vi "_Read.vi"(8 "error in (no error)":errorcluster, 11 "Synapse CCD in":refnum<class "Synapse CCD.lvclass">) -> (0 "error out":errorcluster, 2 "X array":T1, 3 "Synapse CCD out":refnum<class "Synapse CCD.lvclass">)   [LabVIEW 2012, in "Synapse CCD.lvclass"]
doc: "(Protected, Dynamic, Pure Virtual/Abstract) Perform a measurement and return one or more channels of data. Outsiders should not call this method, but instead the public \"Read Data.vi\"."
uses:
  Synapse CCD.lvclass
  Utility Classes/Readable/X array.ctl
  Utility Classes/Readable/X.ctl
  Utility Classes/Readable/Readable.lvclass
  Synapse CCD.lvclass/Synapse CCD.ctl
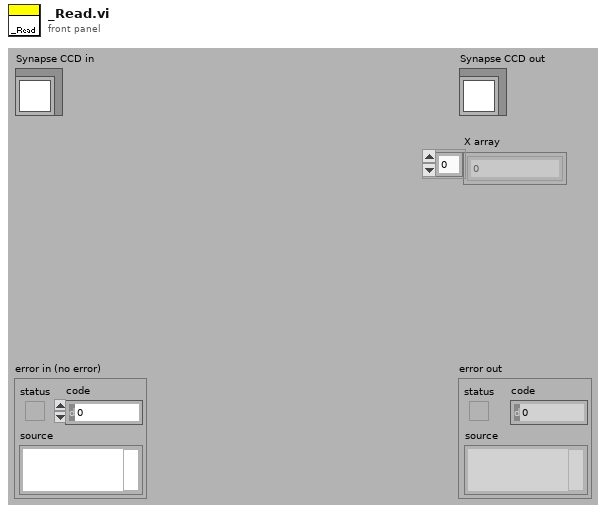
[diagram p1: front panel]
types:
  T1 = typedef "Readable.lvclass/X array.ctl" = T2[]
  T2 = typedef "Readable.lvclass/X.ctl" = dbl
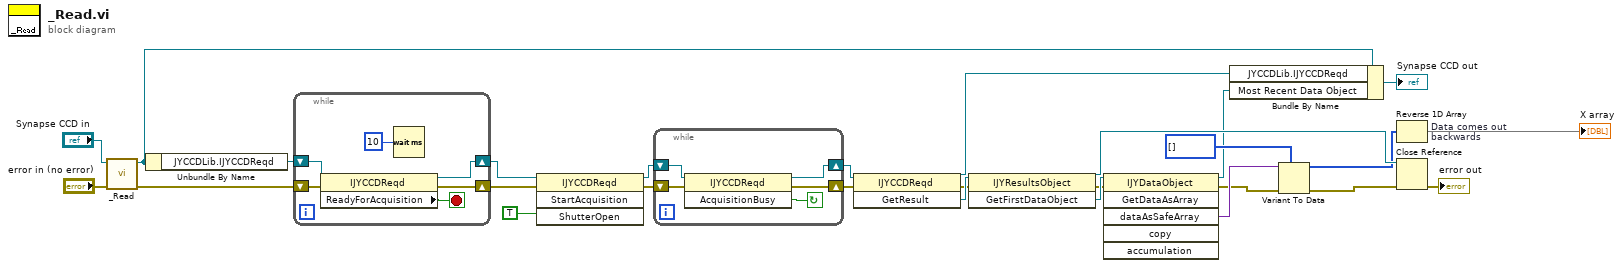
[diagram p0: block diagram]
diagram:
  n1 = call-parent "_Read.vi"("error in (no error)"="error in (no error)", "Readable in"="Synapse CCD in") -> ("error out"=w24:errorcluster, "Readable out"=w17:refnum<class "Synapse CCD.lvclass">)  [unwired: 7 in, 1 out]
  n2 = Unbundle By Name(w17) -> ("JYCCDLib.IJYCCDReqd"=w25:refnum<k7>)
  n3 = while {
    shift-right: [w32] -> w5
    shift-left: w25 -> [w33]
    shift-right: [w30] -> w6
    shift-left: w24 -> [w31]
    stop <- w29 stop-if-true
    n4 = property class="IJYCCDReqd"(reference=w33, error in=w31) -> (reference out=w32:refnum<k7>, error out=w30:errorcluster, "ReadyForAcquisition"=w29:bool)
    n5 = Wait (ms)(milliseconds to wait=u32 10) -> ()  [unwired: 1 out]
  }
  n6 = invoke class="IJYCCDReqd" method="StartAcquisition"(reference=w5, error in=w6, "ShutterOpen"=TRUE) -> (reference out=w23:refnum<k7>, error out=w22:errorcluster)  [unwired: 1 in, 2 out]
  n7 = while {
    shift-right: [w35] -> w3
    shift-left: w23 -> [w38]
    shift-right: [w34] -> w4
    shift-left: w22 -> [w37]
    stop <- w36 continue-if-true
    n8 = invoke class="IJYCCDReqd" method="AcquisitionBusy"(reference=w38, error in=w37) -> (reference out=w35:refnum<k7>, error out=w34:errorcluster, "AcquisitionBusy"=w36:bool)  [unwired: 1 in]
  }
  n9 = invoke class="IJYCCDReqd" method="GetResult"(reference=w3, error in=w4) -> (reference out=w15:refnum<k7>, error out=w13:errorcluster, "GetResult"=w21:refnum<k7>)  [unwired: 1 in]
  n10 = invoke class="IJYResultsObject" method="GetFirstDataObject"(reference=w21, error in=w13) -> (reference out=w14:refnum<k7>, error out=w12:errorcluster, "GetFirstDataObject"=w20:refnum<k7>)  [unwired: 1 in]
  n11 = invoke class="IJYDataObject" method="GetDataAsArray"(reference=w20, error in=w12) -> (reference out=w1:refnum<k7>, error out=w11:errorcluster, "dataAsSafeArray"=w19:variant)  [unwired: 4 in, 3 out]
  n12 = Bundle By Name(cluster=w17, "JYCCDLib.IJYCCDReqd"=w15, "Most Recent Data Object"=w1) -> (→"Synapse CCD out":refnum<class "Synapse CCD.lvclass">)
  n13 = Variant To Data(error in=w11, type=i32[] [], Variant=w19) -> (data=w8:i32[], error out=w10:errorcluster)
  n14 = Reverse 1D Array "Data comes out backwards"(array=w8) -> (reversed array=→"X array":i32[])
  n15 = Close Reference(reference=w14, error in (no error)=w10) -> (error out=→"error out":errorcluster)
